vi "colorchanger.vi"() -> ()   [LabVIEW 2019]
uses:
  <vilib>/LabVIEW Interface for Arduino/Type Defs/Board Type.ctl
  <vilib>/LabVIEW Interface for Arduino/LabVIEW Interface for Arduino.lvlib
panel:
  out "error out":errorcluster
  out "source":string
  out "code":i32
  out "status":bool
  in  "green":dbl
  in  "blue":dbl
  in  "red":dbl
  out "blue":dbl
  out "green":dbl
  out "red":dbl
  in  "Color":u32(colorbox)
  in  "stop":bool
  in  "Blue Pin":u8
  in  "Green Pin":u8
  in  "Red Pin":u8
  in  "VISA resource":refnum<visa-resource-name>
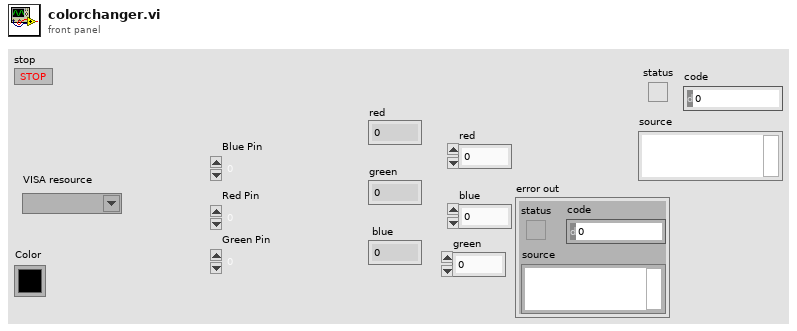
[diagram p1: front panel]
types:
  T1 = typedef "LabVIEW Interface for Arduino.lvlib/Board Type.ctl" = enum16{"Uno", "Dimuelanove w/Atmega 328", "Mega 2560"}
  T2 = typedef "LabVIEW Interface for Arduino.lvlib/Arduino Resource.ctl" = cluster{"VISA resource":refnum<visa-resource-name>, "Board Type":T1, "Connection Type":enum8{"USB / Serial"}, "Bytes Per Packet (15)":u8}
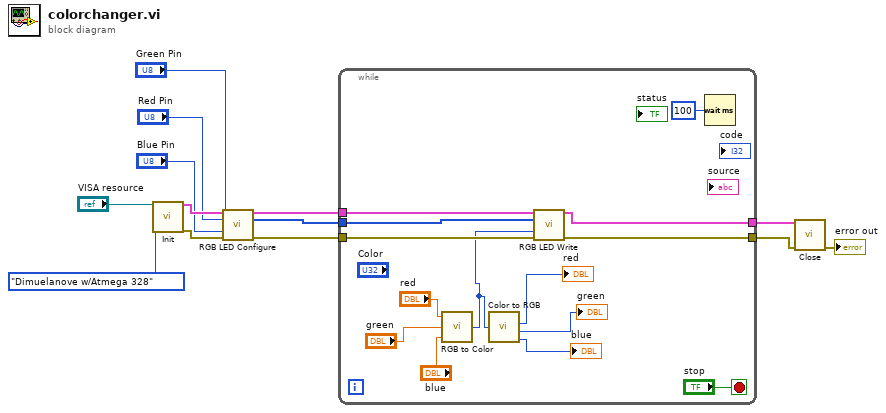
[diagram p0: block diagram]
diagram:
  n1 = call <vilib>:"Init.vi"("VISA resource"="VISA resource", "Board Type (Uno)"=Board_Type."Dimuelanove w/Atmega 328") -> ("Arduino Resource"=w12:T2, "error out"=w11:errorcluster)  [unwired: 16 in]
  n2 = call <vilib>:"RGB LED Configure.vi"("Arduino Resource"=w12, "Red Pin"="Red Pin", "Green Pin"="Green Pin", "Blue Pin"="Blue Pin", "error in"=w11) -> ("Arduino Resource"=w6:T2, "RGB LED Pins"=w4:u8[], "error out"=w5:errorcluster)  [unwired: 8 in]
  n3 = while {
    tunnel: w6 -> [w25]
    tunnel: w5 -> [w24]
    tunnel: w4 -> [w23]
    tunnel: [w22] -> w3
    tunnel: [w21] -> w2
    stop <- "stop" stop-if-true
    n4 = call <vilib>:"RGB to Color.vi"("B"="blue", "G"="green", "R"="red") -> ("Color"=w14:u32)
    n5 = call <vilib>:"Color to RGB.vi"("Color"=w14) -> ("R"=→"red":u8, "G"=→"green":u8, "B"=→"blue":u8)  [unwired: 1 out]
    n6 = call <vilib>:"RGB LED Write.vi"("Arduino Resource"=w25, "RGB LED Pins"=w23, "Color"=w14, "error in"=w24) -> ("Arduino Resource"=w22:T2, "error out"=w21:errorcluster)  [unwired: 9 in, 1 out]
    n7 = Wait (ms)(milliseconds to wait=u32 100) -> ()  [unwired: 1 out]
  }
  n8 = call <vilib>:"Close.vi"("Arduino Resource"=w3, "error in"=w2) -> ("error out"=→"error out":errorcluster)  [unwired: 13 in]
